vi "Build and Parse Data.vi"(0 "SRL Message Out":string, 5 "Cycle Instructions":T1[](array[typedef]) {"Post CMD Delay (s)" format="%#_4ps"; "DAC Vout (V)" format="%.3f V"; "Dev Ch Idx (0-5)" max=5 step=1 format="Ch %d"}, 7 "Clock Rate (Hz) (Cycle Only)":dbl=50000.0, 9 "SRL Data In [U8]":u8[][](array[numeric]) format="%02x", 12 "Simulate FPGA (Cycle Only)":bool, 13 "Dev Mask (All)":bool[](array[boolean])=[TRUE, TRUE, TRUE, TRUE, TRUE, TRUE]) -> (4 "SRL Data Out [U8]":u8[][](array[numeric]) format="%02x", 10 "SRL Message In":string[](array[string]))   [LabVIEW 2017, in "Host SRL.lvlib"]
uses:
  Host SRL.lvlib
  Type Defs/Cycle Instruction Cluster.ctl
panel:
  # "Dev 01"
  # "Dev 02"
  # "Dev 03"
  # "Dev 04"
  # "Dev 05"
  # "Dev 06"
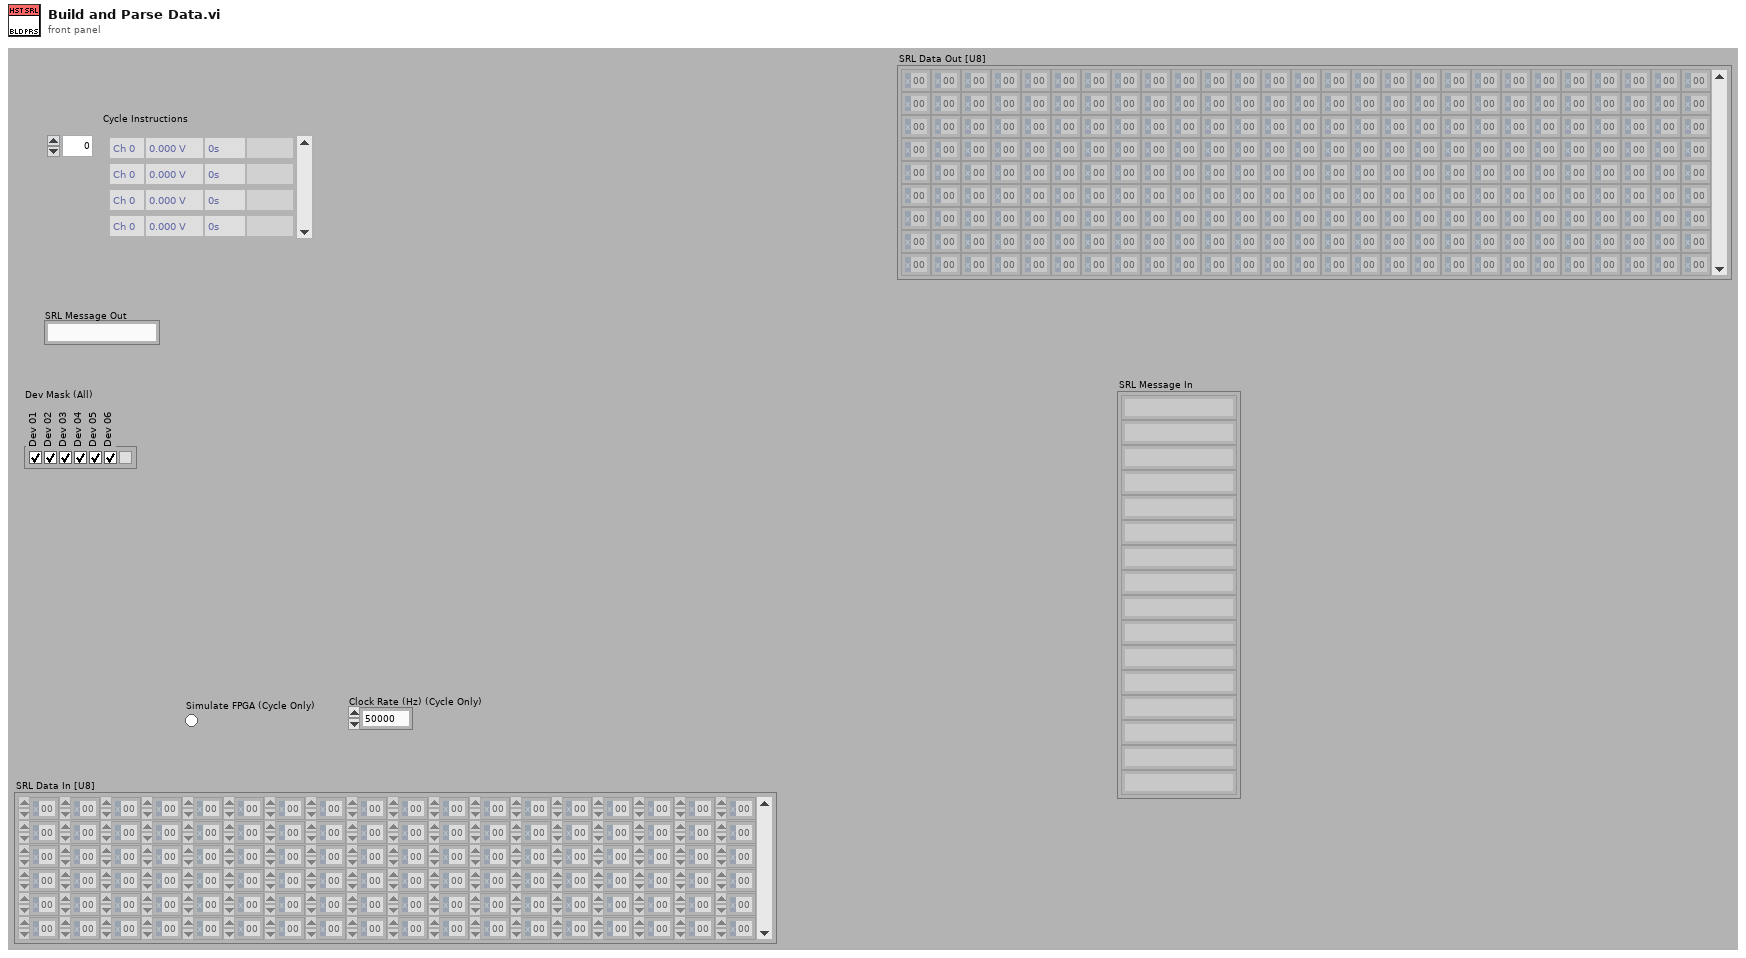
[diagram p1: front panel]
types:
  T1 = typedef "Host SRL.lvlib/Cycle Instruction Cluster.ctl" = cluster{"Dev Ch Idx (0-5)":u32, "DAC Vout (V)":dbl, "Post CMD Delay (s)":dbl, "Raw CMD":string}
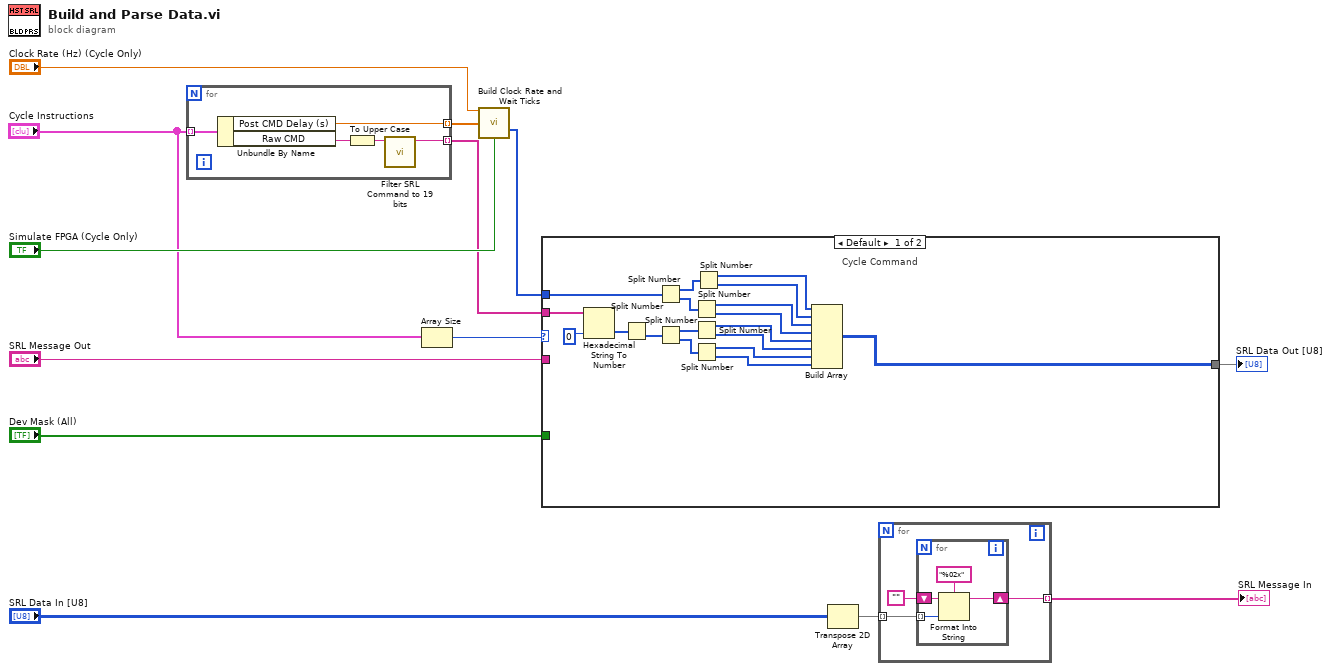
[diagram p0: block diagram]
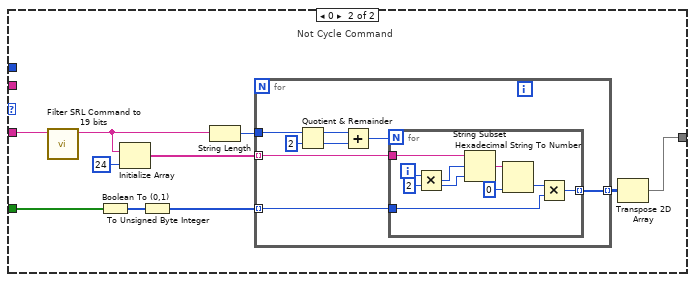
[diagram p2: hidden frame]
diagram:
  n1 = for {
    tunnel: "Cycle Instructions" -> [w18] mode=indexing
    tunnel: [w15] -> w4 mode=indexing
    tunnel: [w14] -> w5 mode=indexing
    n2 = Unbundle By Name(w18) -> ("Post CMD Delay (s)"=w14:dbl, "Raw CMD"=w17:string)
    n3 = To Upper Case(1:w17) -> (0:w16:string)
    n4 = call "Filter SRL Command to 19 bits.vi"("SRL Command In"=w16) -> ("19-bit SRL Command"=w15:string)  [unwired: 10 in]
  }
  n5 = Array Size(array="Cycle Instructions") -> (size(s)=w3:i32)
  n6 = call "Build Clock Rate and Wait Ticks.vi"("Clock Rate (Hz)"="Clock Rate (Hz) (Cycle Only)", "CMD Delay (s)"=w5, "Simulate FPGA"="Simulate FPGA (Cycle Only)") -> ("CMD Delay (Ticks)"=w1:u32[])  [unwired: 9 in, 3 out]
  n7 = case shown="Default" w3 {
    tunnel: "Dev Mask (All)" -> [_ w46]
    tunnel: [w20 w41] -> w10
    tunnel: "SRL Message Out" -> [_ w38]
    tunnel: w4 -> [w36 _]
    tunnel: w1 -> [w19 _]
    frame Default {
      # "Cycle Command"
      n8 = Hexadecimal String To Number(string=w36, default (0uL)=u64 0 ("Read Data")) -> (number=w30:u64[])  [unwired: 1 in, 1 out]
      n9 = Split Number(x=w30) -> (lo(x)=w34:u32[])  [unwired: 1 out]
      n10 = Split Number(x=w19) -> (hi(x)=w23:u16[], lo(x)=w33:u16[])
      n11 = Split Number(x=w34) -> (hi(x)=w32:u16[], lo(x)=w31:u16[])
      n12 = Split Number(x=w33) -> (hi(x)=w24:u8[], lo(x)=w29:u8[])
      n13 = Split Number(x=w32) -> (hi(x)=w28:u8[], lo(x)=w27:u8[])
      n14 = Split Number(x=w31) -> (hi(x)=w26:u8[], lo(x)=w25:u8[])
      n15 = Split Number(x=w23) -> (hi(x)=w21:u8[], lo(x)=w22:u8[])
      n16 = Build Array(w21, w22, w24, w29, w28, w27, w26, w25) -> (w20:u8[][])
    }
    frame 0 {
      # "Not Cycle Command"
      n17 = call "Filter SRL Command to 19 bits.vi"("SRL Command In"=w38) -> ("19-bit SRL Command"=w37:string)  [unwired: 10 in]
      n18 = Boolean To (0,1)(Boolean=w46) -> (0, 1=w45:i16[])
      n19 = Initialize Array(w37, 24 ("dimension size")) -> (w40:string[])
      n20 = To Unsigned Byte Integer(number=w45) -> (unsigned 8bit integer=w44:u8[])
      n21 = String Length(string=w37) -> (length=w39:i32)
      n22 = for {
        tunnel: w44 -> [w53] mode=indexing
        tunnel: [w52] -> w43 mode=indexing
        tunnel: w40 -> [w51] mode=indexing
        tunnel: w39 -> [w50]
        n23 = Quotient & Remainder(x=w50, y=2) -> (x-y*floor(x/y)=w49:i32, floor(x/y)=w48:i32)
        n24 = Add(x=w49, y=w48) -> (x+y=w47:i32)
        n25 = for {
          N: w47 -> [_]
          tunnel: w51 -> [w63]
          tunnel: [w56] -> w52 mode=indexing
          tunnel: w53 -> [w57]
          i -> [w62]
          w60 = 2 ("y")
          n26 = Multiply(x=w62, y=w60) -> (x*y=w61:i32)
          n27 = String Subset(string=w63, offset (0)=w61, length (rest)=w60) -> (substring=w59:string)
          n28 = Hexadecimal String To Number(string=w59, default (0uL)=u8 0 ("default (0 U32)")) -> (number=w55:u8)  [unwired: 1 in, 1 out]
          n29 = Multiply(x=w55, y=w57) -> (x*y=w56:u8)
        }
      }
      n30 = Transpose 2D Array(2D array=w43) -> (transposed array=w41:u8[][])
    }
  }
  "SRL Data Out [U8]" <- w10
  n31 = Transpose 2D Array(2D array="SRL Data In [U8]") -> (transposed array=w12:u8[][])
  n32 = for {
    tunnel: w12 -> [w66] mode=indexing
    tunnel: [w64] -> w11 mode=indexing
    n33 = for {
      tunnel: w66 -> [w70] mode=indexing
      shift-right: [w68] -> w64
      shift-left: "" -> [w67]
      n34 = Format Into String(format string="%02x", initial string=w67, w70) -> (resulting string=w68:string)  [unwired: 1 in, 1 out]
    }
  }
  "SRL Message In" <- w11
